vi "Choose_Many_Folders.vi"(1 "Purpose of choosing folder":string) -> (0 "Files":path[](array[path]))   [LabVIEW 2010]
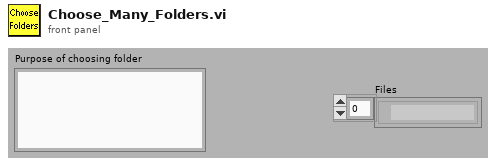
[diagram p1: front panel]
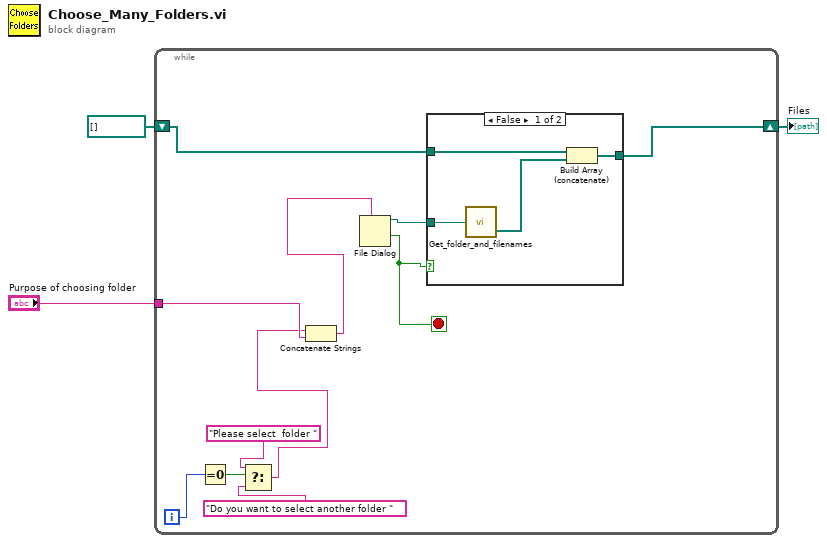
[diagram p0: block diagram]
diagram:
  n1 = while {
    shift-right: [w5] -> w1
    shift-left: path[] [] -> [w6]
    tunnel: "Purpose of choosing folder" -> [w10]
    i -> [w14]
    stop <- w4 stop-if-true
    n2 = Equal To 0?(x=w14) -> (x = 0?=w13:bool)
    n3 = Select(t="Please select  folder " ("prompt"), s=w13, f="Do you want to select another folder " ("prompt")) -> (s? t:f=w9:string)
    n4 = Concatenate Strings(w9, w10) -> (w8:string)
    n5 = File Dialog(7:w8) -> (1:w4:bool, 3:w7:path)  [unwired: 6 in, 2 out]
    n6 = case shown="False" w4 {
      tunnel: w7 -> [w18 _]
      tunnel: w6 -> [w17 w19]
      tunnel: [w15 w19] -> w5
      frame False {
        n7 = call "Get_folder_and_filenames.vi"("file path (dialog if empty)"=w18) -> ("Files"=w16:path[])  [unwired: 1 out]
        n8 = Build Array (concatenate)(w17, w16) -> (w15:path[])
      }
      frame True {
      }
    }
  }
  "Files" <- w1
